vi "Refresh Values.vi"(8 "error in (no error)":errorcluster, 11 "PluginGUI in":refnum<class "PluginGUI.lvclass">) -> (0 "error out":errorcluster, 3 "PluginGUI out":refnum<class "PluginGUI.lvclass">)   [LabVIEW 2020, in "VolatusGUI.lvlib" / "PluginGUI.lvclass"]
uses:
  PluginGUI.lvclass
  PluginGUI.lvclass/PluginGUI.ctl
  GUI Element/GUI Element.lvclass
  Volatus/Module/Module.lvclass
  C:/dev/lv20CE/relink/lv-volatus/Volatus/Module/Module.lvclass
  C:/dev/lv20CE/relink/lv-volatus/VolatusGUI/PluginGUI/PluginGUI.lvclass
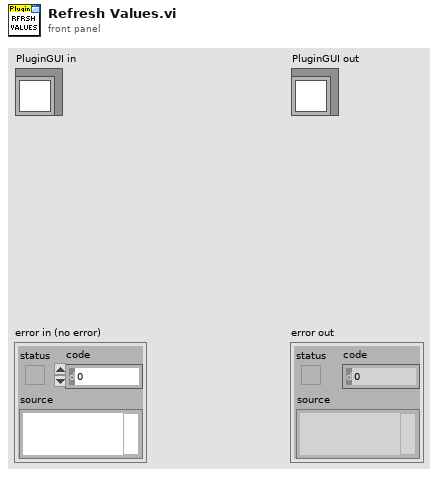
[diagram p1: front panel]
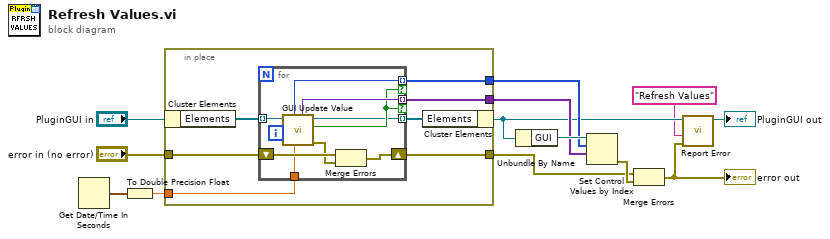
[diagram p0: block diagram]
diagram:
  n1 = Get Date/Time In Seconds() -> (seconds since 1Jan1904=w3:timestamp)
  n2 = To Double Precision Float(number=w3) -> (double precision float=w2:dbl)
  n3 = in-place {
    in-place-border: "error in (no error)" -> [w20]
    in-place-border: [w19] -> w11
    in-place-border: [w18] -> w10
    in-place-border: [w14] -> w6
    in-place-border: w2 -> [w15]
    n4 = in-place-cluster #1("PluginGUI in") -> ("Elements"=w17:refnum<class "GUI Element.lvclass">[])
    n5 = for {
      tunnel: [w26] -> w19 mode=indexing if=w24
      tunnel: [w25] -> w18 mode=indexing if=w24
      shift-right: [w27] -> w14
      shift-left: w20 -> [w29]
      tunnel: w17 -> [w23] mode=indexing
      tunnel: [w22] -> w16 mode=indexing
      tunnel: w15 -> [w21]
      n6 = call "GUI Update Value.vi"("Time"=w21, "GUI Element in"=w23) -> ("error out"=w28:errorcluster, "Update"=w24:bool, "GUI Element out"=w22:refnum<class "GUI Element.lvclass">, "Value"=w25:variant, "Control Index"=w26:i32)  [unwired: 5 in]
      n7 = Merge Errors(w29, w28) -> (w27:errorcluster)
    }
    n8 = in-place-cluster #1("Elements"=w16) -> (w5:refnum<class "PluginGUI.lvclass">)
  }
  n9 = Unbundle By Name(w5) -> ("GUI"=w12:refnum<vi>)
  n10 = Set Control Values by Index(0:w12, 1:w11, 2:w10) -> (11:w9:errorcluster)  [unwired: 1 in]
  n11 = Merge Errors(w6, w9) -> (w8:errorcluster)
  "error out" <- w8
  n12 = call "Report Error.vi"("error in (no error)"=w8, "Message (None)"="Refresh Values", "Module in"=w5) -> ("Module out"=→"PluginGUI out":refnum<class "PluginGUI.lvclass">)  [unwired: 7 in, 1 out]
